vi "Create.vi"(5 "Binary Operator in":refnum<class "Binary Operator.lvclass">, 8 "error in (no error)":errorcluster, 11 "Constraints":refnum<class "Constraint.lvclass">[](array[class])) -> (0 "error out":errorcluster, 3 "Binary Operator":refnum<class "Binary Operator.lvclass">)   [LabVIEW 2017, in "Transparent Assertions.lvlib" / "Constraints.lvlib" / "Binary Operator.lvclass"]
uses:
  Binary Operator.lvclass
  Constraint/Constraint.lvclass
  Binary Operator.lvclass/Binary Operator.ctl
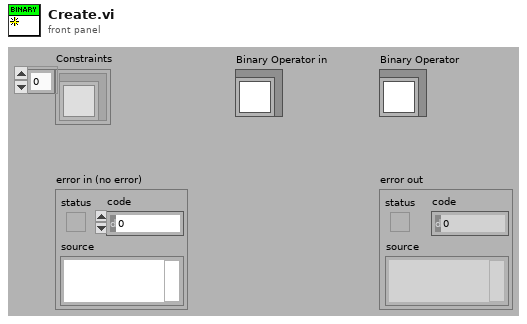
[diagram p1: front panel]
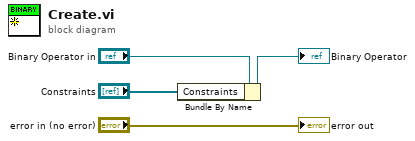
[diagram p0: block diagram]
diagram:
  n1 = Bundle By Name(cluster="Binary Operator in", "Constraints"="Constraints") -> (→"Binary Operator":refnum<class "Binary Operator.lvclass">)
  "error out" <- "error in (no error)"
